vi "CfgUI.vi"(7 "LabVIEW Web Service Request":refnum<class "Web Request.lvclass">) -> ()   [LabVIEW 2014]
doc: "Call this web service to poll for changes in control values generated on the embedded system rather than at the user interface."
uses:
  <vilib>/wsapi/Web Request.lvclass
  Controller/Controls/Notifier Enum.ctl
  Controller/Controller.lvclass
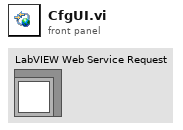
[diagram p1: front panel]
types:
  T1 = typedef "Controller.lvlib/Controller.lvclass/Notifier Enum.ctl" = enum16{"Initialize", "Get", "Set", "Close"}
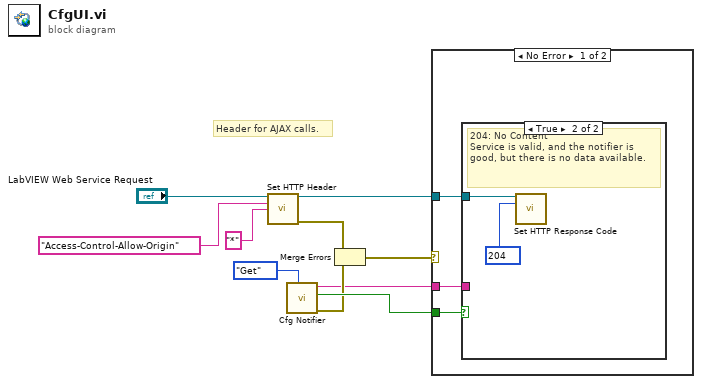
[diagram p0: block diagram]
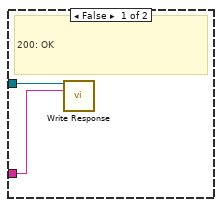
[diagram p2: hidden frame]
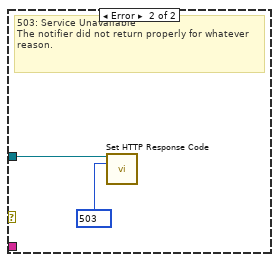
[diagram p3: hidden frame]
diagram:
  # "Header for AJAX calls."
  n1 = call <vilib>:"Set HTTP Header.vi"("LabVIEW Web Service Request"="LabVIEW Web Service Request", "header"="Access-Control-Allow-Origin", "header value"="*") -> ("LabVIEW Web Service Request out"=w6:refnum<class "Web Request.lvclass">, "error out"=w4:errorcluster)  [unwired: 11 in]
  n2 = call "Cfg Notifier.vi"("State"=Notifier_Enum."Get") -> ("error out"=w5:errorcluster, "timed out?"=w8:bool, "Data Out"=w3:string)  [unwired: 8 in]
  n3 = Merge Errors(w4, w5) -> (w2:errorcluster)
  n4 = case shown="No Error" w2 {
    tunnel: w8 -> [w13 _]
    tunnel: w6 -> [w12 w19]
    tunnel: w3 -> [w11 _]
    frame No Error {
      n5 = case shown="True" w13 {
        tunnel: w12 -> [w15 w17]
        tunnel: w11 -> [w14 _]
        frame False {
          # "200: OK"
          n6 = call <vilib>:"Write Response.vi"("LabVIEW Web Service Request"=w15, "response string"=w14) -> ()  [unwired: 12 in, 2 out]
        }
        frame True {
          w16 = 204 items=["100"=100, "101"=101, "200"=200, "201"=201, "202"=202, "203"=203, "204"=204, "205"=205, "206"=206, "300"=300, "301"=301, "302"=302, "303"=303, "304"=304, "305"=305, "306"=306, "307"=307, "400"=400, "401"=401, "402"=402, "403"=403, "404"=404, "405"=405, "406"=406, "407"=407, "408"=408, "409"=409, "410"=410, "411"=411, "412"=412, "413"=413, "414"=414, "415"=415, "416"=416, "417"=417, "500"=500, "501"=501, "502"=502, "503"=503, "504"=504, "505"=505] ("response code (200)")
          # "204: No Content\nService is valid, and the notifier is good, but there is no data available."
          n7 = call <vilib>:"Set HTTP Response Code.vi"("LabVIEW Web Service Request"=w17, "response code (200)"=w16) -> ()  [unwired: 12 in, 2 out]
        }
      }
    }
    frame Error {
      w18 = 503 items=["100"=100, "101"=101, "200"=200, "201"=201, "202"=202, "203"=203, "204"=204, "205"=205, "206"=206, "300"=300, "301"=301, "302"=302, "303"=303, "304"=304, "305"=305, "306"=306, "307"=307, "400"=400, "401"=401, "402"=402, "403"=403, "404"=404, "405"=405, "406"=406, "407"=407, "408"=408, "409"=409, "410"=410, "411"=411, "412"=412, "413"=413, "414"=414, "415"=415, "416"=416, "417"=417, "500"=500, "501"=501, "502"=502, "503"=503, "504"=504, "505"=505] ("response code (200)")
      # "503: Service Unavailable\nThe notifier did not return properly for whatever reason."
      n8 = call <vilib>:"Set HTTP Response Code.vi"("LabVIEW Web Service Request"=w19, "response code (200)"=w18) -> ()  [unwired: 12 in, 2 out]
    }
  }
